vi "Get HTTP Port.vi"(8 "error in (no error)":errorcluster, 11 "Node Config in":refnum<class "Node Config.lvclass">) -> (0 "error out":errorcluster, 2 "HTTP Port":u16, 3 "Node Config out":refnum<class "Node Config.lvclass">)   [LabVIEW 2020, in "VolatusConfig.lvlib" / "Node Config.lvclass"]
uses:
  Node Config.lvclass
  Node Config.lvclass/Node Config.ctl
  VolatusConfigElement/VolatusConfigElement.lvclass
  lv-cdm/CDM-Config/Config Element/Config Element.lvclass
  C:/dev/lv20CE/relink/lv-volatus/VolatusConfig/VolatusConfigElement/VolatusConfigElement.lvclass
  C:/dev/lv20CE/relink/lv-volatus/VolatusConfig/Node/Node Config.lvclass
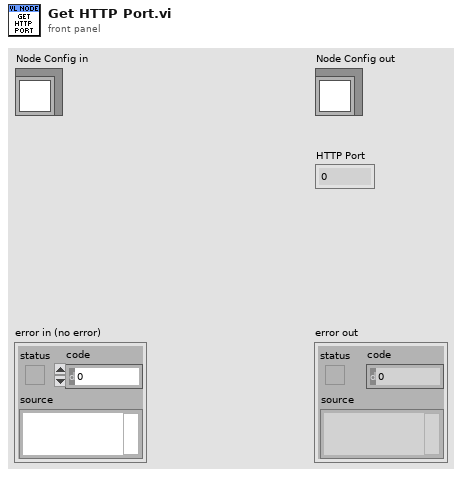
[diagram p1: front panel]
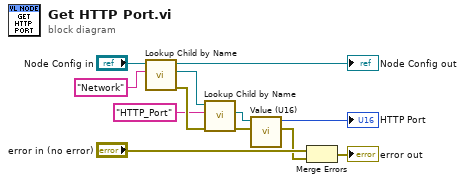
[diagram p0: block diagram]
diagram:
  n1 = call "Lookup Child by Name.vi"("Child Name"="Network", "VolatusConfigElement in"="Node Config in") -> ("error out"=w7:errorcluster, "Child"=w8:refnum<class "Config Element.lvclass">, "VolatusConfigElement out"=→"Node Config out":refnum<class "Node Config.lvclass">)  [unwired: 6 in, 1 out]
  n2 = call "Lookup Child by Name.vi"("error in (no error)"=w7, "Name"="HTTP_Port", "Config Element in"=w8) -> ("error out"=w5:errorcluster, "Child"=w4:refnum<class "Config Element.lvclass">)  [unwired: 5 in, 2 out]
  n3 = call "Value (U16).vi"("error in (no error)"=w5, "Config Element in"=w4) -> ("error out"=w1:errorcluster, "U16 Value"=→"HTTP Port":u16)  [unwired: 8 in]
  n4 = Merge Errors("error in (no error)", w1) -> (→"error out":errorcluster)
